vi "5_7.vi"() -> ()   [LabVIEW 2017]
panel:
  in  "Array":dbl[](array[numeric])
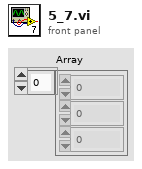
[diagram p1: front panel]
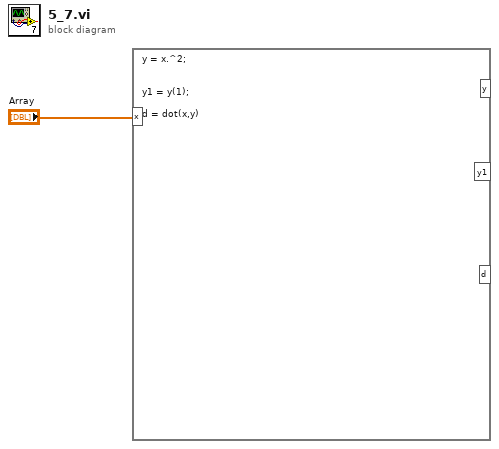
[diagram p0: block diagram]
diagram:
  n1 = formula code="y = x.^2;\n\n\ny1 = y(1);\n\nd = dot(x,y)"("x"="Array") -> ()  [unwired: 1 in, 2 out]
